vi "Load File Preview.vi"(4 "Y-Array":dbl[](array[numeric]) format="%.2f", 5 "X-Array":dbl[](array[numeric]) format="%.2f", 7 "File Contents":string, 9 "File Path":path) -> (0 "Continue?":bool, 2 "WL unit copy":i32(ring)=1 items=["Wavelength", "nm", "eV", "meV", "cm-1"], 3 "File Parameter Out":T1={"FilePath"=path "/DATA/Labview Items", "Field (T)"=55.0, "Temperature (K)"=77.0, "X-Axis"=enum."nm", "Center nm"=55.0, "Current Grating Density"=enum."600", "CCD Parameters"={"Exposure Time (s)"=0.2, "Offset"=0.0, "BkgrdCrct"=FALSE, "Shutter"=FALSE, "Mode"=enum."Regular", "Repetition"=4, "dt or s"=0.0}, "Operation Mode"=enum."NML Data Acquisition", "Exp Index"=0, "Index_repetition"=0, "Index"=0, "Current Detector"=enum."CCD-1024x256"} {"CCD Parameters"."dt or s" format="%#.6f"; "CCD Parameters"."Repetition" min=1; "CCD Parameters"."Offset" format="%#.2f"; "CCD Parameters"."Exposure Time (s)" min=0.02 max=6000.0 format="%#.2f"; "Center nm" format="%.2f"; "Temperature (K)" format="%.2f"; "Field (T)" format="%.2f"})   [LabVIEW 2020]
uses:
  Globals and TypeDefs/Type Definitions.llb/FileInfoParameter.ctt
  Globals and TypeDefs/Type Definitions.llb/Wavelength Unit.ctt
  Globals and TypeDefs/Type Definitions.llb/McPherson Grating Density.ctl
  Globals and TypeDefs/Type Definitions.llb/CCDParameter.ctt
  Globals and TypeDefs/Type Definitions.llb/OperationMode.ctt
  Globals and TypeDefs/Type Definitions.llb/ListOfDetectors.ctt
  Globals and TypeDefs/gDetector.vi
  File and save/X-Axis Converter.llb/X-Axis Converter.vi
  File and save/X-Axis_Generator_x.vi
panel:
  in  "Grating Density":enum16{"150", "300", "600", "1200", "1800"}(ring)
  in  "Center nm":dbl format="%.2f"
  in  "Temperature (K)":dbl format="%.2f"
  in  "Field (T)":dbl format="%.2f"
  out "?":T7(graph)
  in  "Cancel":bool
  in  "Continue?":bool
  in  "WL unit":i32(ring)=1 items=["Wavelength", "nm", "eV", "meV", "cm-1"]
  # "Please double check the file,\nif it contains valid data, \nselect the wavelength unit \nUSED IN THE FILE:"
  # "Hit \"OK\" to load the data\nor \"Cancel\" to abort."
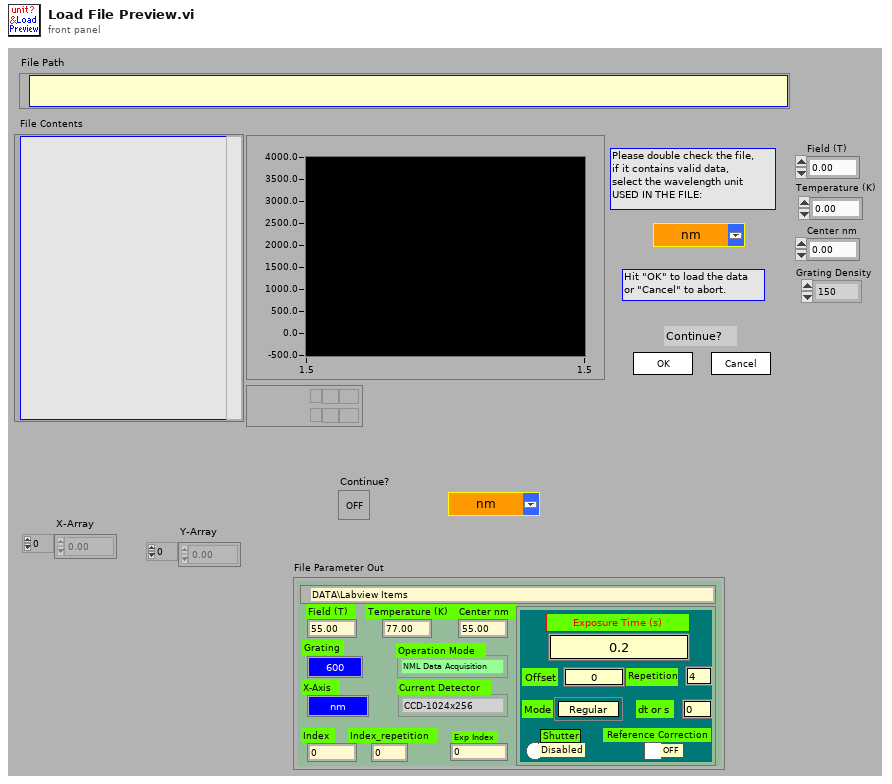
[diagram p1: front panel]
types:
  T1 = typedef "FileInfoParameter.ctt" = cluster{"FilePath":path, "Field (T)":dbl, "Temperature (K)":dbl, "X-Axis":T2, "Center nm":dbl, "Current Grating Density":T3, "CCD Parameters":T4, "Operation Mode":T5, "Exp Index":u32, "Index_repetition":u16, "Index":u16, "Current Detector":T6}
  T2 = typedef "Wavelength Unit.ctt" = enum8{"Point", "nm", "eV", "meV", "cm_1"}
  T3 = typedef "McPherson Grating Density.ctl" = enum8{"150", "300", "600", "1200", "1800"}
  T4 = typedef "CCDParameter.ctt" = cluster{"Exposure Time (s)":dbl, "Offset":dbl, "BkgrdCrct":bool, "Shutter":bool, "Mode":enum8{"Regular", "OverExp Cor", "SpikeRemove", "ForCalibration"}, "Repetition":u16, "dt or s":dbl}
  T5 = typedef "OperationMode.ctt" = enum16{"Standby", "CCD Single Shot", "CCD Sequence Shots", "CCD Custom Shots", "CCD Reference Shot", "Step Scanning ", "Time Scanning", "NML Data Acquisition"}
  T6 = typedef "ListOfDetectors.ctt" = enum8{"CCD-1024x256", "InGaAs PDA-1024x1", "CCD-1340x400", "Ge Single Channel", "Si Single Channel", "PMT Single Channel"}
  T7 = cluster{"Ramp Pattern":dbl[], "Sinc Pattern":dbl[]}
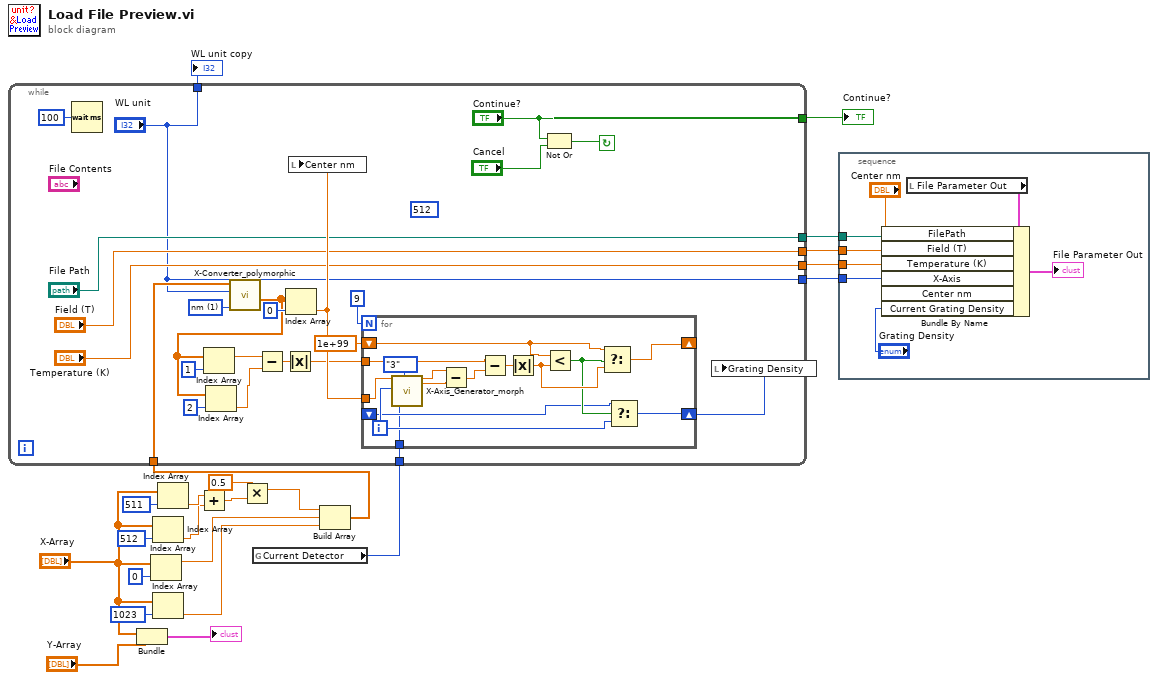
[diagram p0: block diagram]
diagram:
  n1 = Bundle("X-Array"="X-Array", "Y-Array"="Y-Array") -> (→"?":cluster{"X-Array":dbl[], "Y-Array":dbl[]})  [unwired: 1 in]
  n2 = Index Array(array="X-Array", index=0) -> (element=w15:dbl)
  n3 = Index Array(array="X-Array", index=512) -> (element=w5:dbl)
  n4 = Index Array(array="X-Array", index=1023) -> (element=w14:dbl)
  n5 = Index Array(array="X-Array", index=511) -> (element=w6:dbl)
  n6 = Add(x=w6, y=w5) -> (x+y=w3:dbl)
  n7 = Multiply(x=0.5, y=w3) -> (x*y=w4:dbl)
  n8 = global read "gDetector.vi" "Current Detector"() -> (w1:T6)
  n9 = Build Array(w4, w15, w14) -> (w13:dbl[])
  n10 = while {
    tunnel: ["Continue?"] -> w21
    tunnel: ["WL unit"] -> w22
    tunnel: w13 -> [w41]
    tunnel: ["File Path"] -> w12
    tunnel: ["Field (T)"] -> w11
    tunnel: ["Temperature (K)"] -> w10
    tunnel: ["WL unit"] -> w9
    tunnel: w1 -> [w23]
    stop <- w45 continue-if-true
    (unwired) 512 ("X-axis devision")
    w40 = 1 items=["Point #", "nm", "eV", "meV", "cm-1"] ("X-Axis Unit")
    n11 = Wait (ms)(milliseconds to wait=u32 100) -> ()  [unwired: 1 out]
    n12 = call-poly "X-Converter_polymorphic.vi"("X-Axis Unit"=w40, "Old X-Axis Unit"="WL unit", "X-Axis input"=w41) -> ("X-Axis Output"=w36:dbl[])  [unwired: 2 in, 3 out]
    n13 = Index Array(array=w36, index=1) -> (element=w33:dbl)
    n14 = Index Array(array=w36, index=2) -> (element=w32:dbl)
    n15 = Subtract(x=w33, y=w32) -> (x-y=w31:dbl)
    n16 = Absolute Value(x=w31) -> (abs(x)=w30:dbl)
    n17 = Index Array(array=w36, index=0) -> (element=w38:dbl)
    n18 = local write "Center nm"(w38) -> ()
    n19 = for {
      N: 9 -> [_]
      tunnel: w38 -> [w47]
      tunnel: w30 -> [w57]
      shift-right: [w52] -> _
      shift-left: 1e+99 -> [w53]
      shift-right: [w50] -> w28
      shift-left: _ -> [w49]
      tunnel: w23 -> [w46]
      i -> [w60]
      n20 = call-poly "X-Axis_Generator_morph.vi"("Central Wavelength"=w47, "Current Grating Density"=w60, "Current Detector"=w46, "X-Axis Points"=enum16{"1024", "512", "3"}."3") -> ("nm (Max)"=w59:dbl, "nm (Min)"=w58:dbl)  [unwired: 8 in, 6 out]
      n21 = Subtract(x=w59, y=w58) -> (x-y=w56:dbl)
      n22 = Subtract(x=w57, y=w56) -> (x-y=w55:dbl)
      n23 = Absolute Value(x=w55) -> (abs(x)=w54:dbl)
      n24 = Less?(x=w53, y=w54) -> (x < y?=w51:bool)
      n25 = Select(t=w53, s=w51, f=w54) -> (s? t:f=w52:dbl)
      n26 = Select(t=w49, s=w51, f=w60) -> (s? t:f=w50:i32)
    }
    n27 = Not Or(1:"Cancel", 2:"Continue?") -> (0:w45:bool)
    n28 = local write "Grating Density"(w28) -> ()
  }
  "WL unit copy" <- w22
  "Continue?" <- w21
  n29 = stacked-sequence {
    tunnel: w12 -> [w67]
    tunnel: w11 -> [w66]
    tunnel: w10 -> [w65]
    tunnel: w9 -> [w64]
    frame #0 {
      n30 = local read "File Parameter Out"() -> (w68:T1)
      n31 = Bundle By Name(cluster=w68, "FilePath"=w67, "Field (T)"=w66, "Temperature (K)"=w65, "X-Axis"=w64, "Center nm"="Center nm", "Current Grating Density"="Grating Density") -> (→"File Parameter Out":T1)
    }
  }
